vi "Teleop.vi"(10 "Match Info":T2={"Autonomous Elapsed Seconds"=0.0, "TeleOp Elapsed Seconds"=0.0, "Disabled Elapsed Seconds"=0.0, "Visited Autonomous"=FALSE, "Visited TeleOp"=FALSE, "Visited Disabled"=FALSE, "Autonomous Settings"={"Autonomous Style"=enum."Independent", "VI Refnum"=refnum}}, 11 "Call Context":T3) -> ()   [LabVIEW 2019]
doc: "This VI is called for each TeleOp packet received from the DS where the robot is not disabled. It is often used to read from the joysticks and update I/O or to update setpoints for timed control loops. It should complete and return within 20 milliseconds or it may miss DS packets."
uses:
  <vilib>/Rock Robotics/WPI/DriverStation/WPI_DriverStationDerivedRobotMode.ctl
  <vilib>/Rock Robotics/WPI/DriverStation/WPI_DriverStationMatch Info.ctl
  <vilib>/Rock Robotics/WPI/ThirdParty/Phoenix-LabVIEW/Motor Controller/Controls/CTRE_Phoenix_MotorControl_ControlMode.ctl
  <vilib>/Rock Robotics/WPI/Solenoid/WPI_SolenoidValue.ctl
  <vilib>/Rock Robotics/Network Tables/NT Read Boolean.vi
  <vilib>/Rock Robotics/Network Tables/NT Read Number.vi
  <vilib>/Rock Robotics/WPI/Utilities/WPI_GetSetVariantRefNum.vi
  <vilib>/addons/control/pid/pid.llb/PID Output Rate Limiter (DBL).vi
  <vilib>/Rock Robotics/Network Tables/NT Write Numeric Array.vi
  <vilib>/Rock Robotics/Network Tables/NT Write Boolean Array.vi
  <vilib>/Rock Robotics/WPI/Solenoid/WPI_SolenoidSetEnum.vi
  <vilib>/addons/control/pid/NI_PID_pid.lvlib
panel:
  in  "Control Panel":T1 items=["PercentOutput"=0, "Position"=1, "Velocity"=2, "Current"=3, "Follower"=5, "MotionProfile"=6, "MotionMagic"=7, "MotionProfileArc"=10, "Disabled"=15]
  in  "Climber":T1 items=["PercentOutput"=0, "Position"=1, "Velocity"=2, "Current"=3, "Follower"=5, "MotionProfile"=6, "MotionMagic"=7, "MotionProfileArc"=10, "Disabled"=15]
  in  "Outtake":T1 items=["PercentOutput"=0, "Position"=1, "Velocity"=2, "Current"=3, "Follower"=5, "MotionProfile"=6, "MotionMagic"=7, "MotionProfileArc"=10, "Disabled"=15]
  in  "Intake":T1 items=["PercentOutput"=0, "Position"=1, "Velocity"=2, "Current"=3, "Follower"=5, "MotionProfile"=6, "MotionMagic"=7, "MotionProfileArc"=10, "Disabled"=15]
  out "Sample Slider 0":dbl(slide) scale=0.0..5.0
  out "Sample Boolean 1":bool
  out "Sample Boolean 0":bool
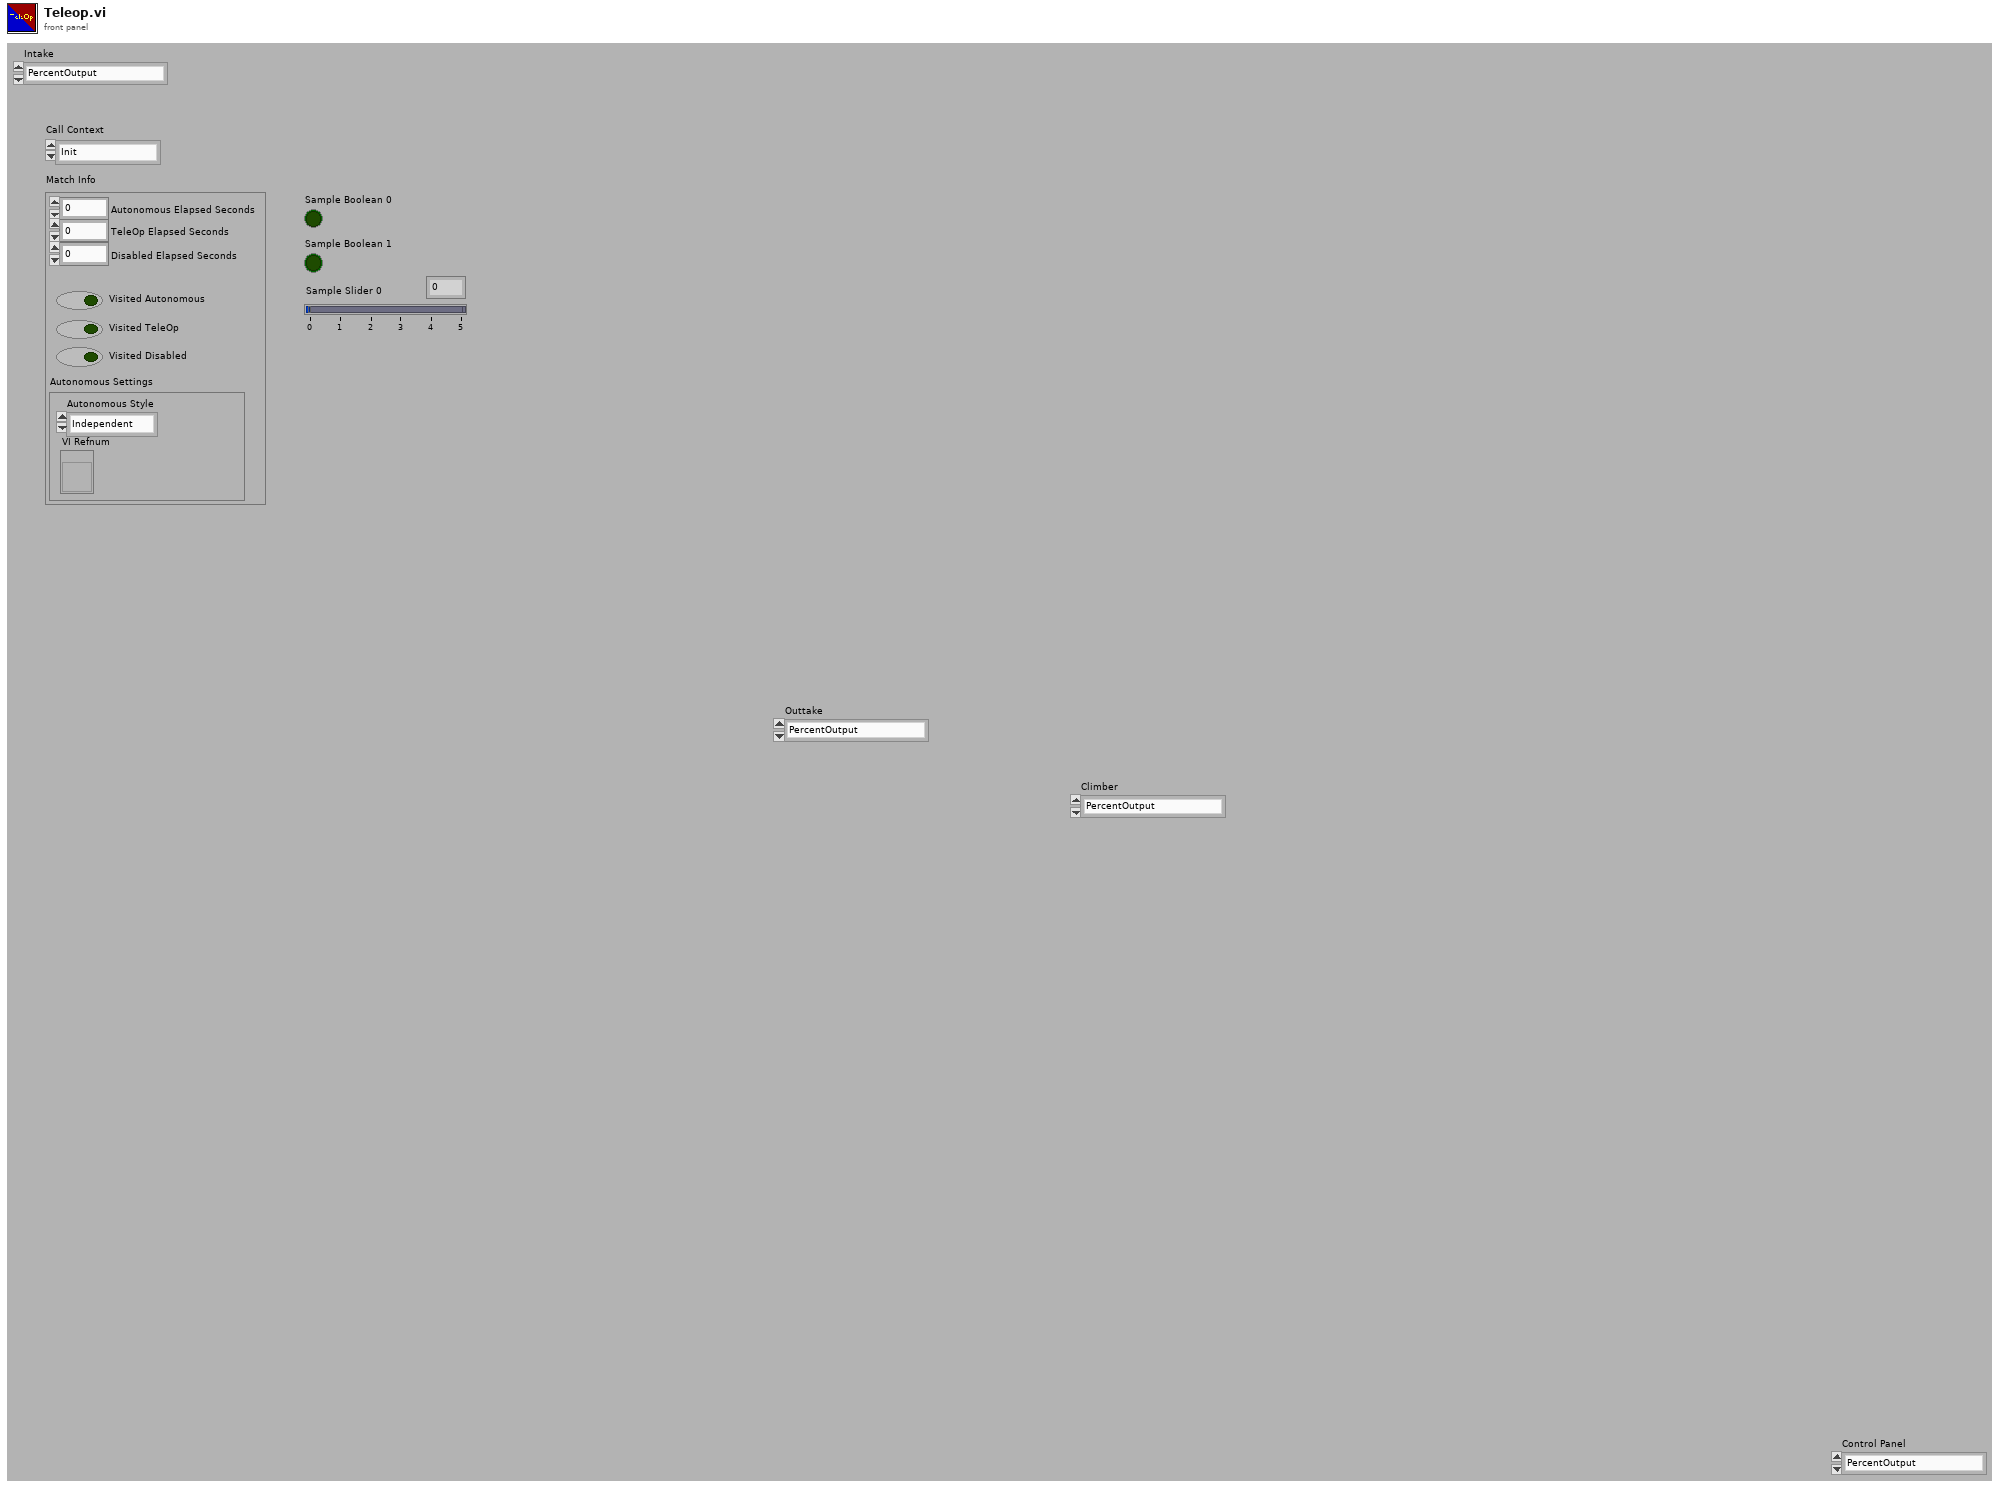
[diagram p1: front panel]
types:
  T1 = typedef "CTRE_Phoenix_MotorControl_ControlMode.ctl" = u16
  T2 = typedef "WPI_DriverStationMatch Info.ctl" = cluster{"Autonomous Elapsed Seconds":dbl, "TeleOp Elapsed Seconds":dbl, "Disabled Elapsed Seconds":dbl, "Visited Autonomous":bool, "Visited TeleOp":bool, "Visited Disabled":bool, "Autonomous Settings":cluster{"Autonomous Style":enum16{"Iterative", "Independent"}, "VI Refnum":refnum<vi>}}
  T3 = typedef "WPI_DriverStationDerivedRobotMode.ctl" = enum16{"Init", "Execute", "Stop"}
  T4 = typedef "WPI_SolenoidValue.ctl" = enum16{"Off", "On", "Forward", "Reverse"}
  T5 = typedef "WPI_RobotDriveDevRef.ctl" = cluster{"DevStatus":errorcluster, "Motors[]":T6[], "Square Inputs":bool, "Max Output":dbl}
  T6 = typedef "WPI_MotorControlDeviceRef.ctl" = cluster{"DeviceStatus":errorcluster, "Type":T7, "PWM":cluster{"PWM Channel":T8, "DeadBand":T9}, "CAN":cluster{"Device Number":u8, "SetOutput VI Ref":variant, "GetOutput VI Ref":variant, "Enable VI Ref":variant, "Disable VI Ref":variant, "Data":variant}, "Invert":bool, "DIO PWM":cluster{"PWM \"Enable\" Channel":T8, "DIOChannel":T10, "PWM Rate":dbl}}
  T7 = typedef "WPI_MotorControlType.ctl" = enum16{"PWM", "CAN", "DIO PWM"}
  T8 = typedef "FPGA_DIOPWMChannel.ctl" = enum8{"PWM 0", "PWM 1", "PWM 2", "PWM 3", "PWM 4", "PWM 5", "PWM 6", "PWM 7", "PWM 8", "PWM 9", "PWM MXP 0", "PWM MXP 1", "PWM MXP 2", "PWM MXP 3", "PWM MXP 4", "PWM MXP 5", "PWM MXP 6", "PWM MXP 7", "PWM MXP 8", "PWM MXP 9", "Invalid"}
  T9 = typedef "WPI_PWMDeadband.ctl" = cluster{"Name":string, "maxPositivePwm":i32, "minPositivePwm":i32, "centerPwm":i32, "maxNegativePwm":i32, "minNegativePwm":i32, "angularRange":u16}
  T10 = typedef "FPGA_DIOChannel.ctl" = enum8{"DIO 0", "DIO 1", "DIO 2", "DIO 3", "DIO 4", "DIO 5", "DIO 6", "DIO 7", "DIO 8", "DIO 9", "DIO MXP 0", "DIO MXP 1", "DIO MXP 2", "DIO MXP 3", "DIO MXP 4", "DIO MXP 5", "DIO MXP 6", "DIO MXP 7", "DIO MXP 8", "DIO MXP 9", "DIO MXP 10", "DIO MXP 11", "DIO MXP 12", "DIO MXP 13", "DIO MXP 14", "DIO MXP 15", "SPI Port CS1", "SPI Port CS2", "SPI Port CS3", "SPI Port MISO", "SPI Port MOSI", "Invalid"}
  T11 = typedef "WPI_JoystickDevRef.ctl" = cluster{"Device":T12}
  T12 = typedef "WPI_JoystickDeviceEnum.ctl" = enum16{"USB 0", "USB 1", "USB 2", "USB 3", "USB 4", "USB 5"}
  T13 = typedef "WPI_SolenoidDevRef.ctl" = cluster{"DevStatus":errorcluster, "Pneumatics Control Module":u8, "Forward Solenoid Channel":T14, "Reverse Solenoid Channel":T14}
  T14 = typedef "WPI_SolenoidChannel.ctl" = enum8{"Solenoid 0", "Solenoid 1", "Solenoid 2", "Solenoid 3", "Solenoid 4", "Solenoid 5", "Solenoid 6", "Solenoid 7", "Invalid"}
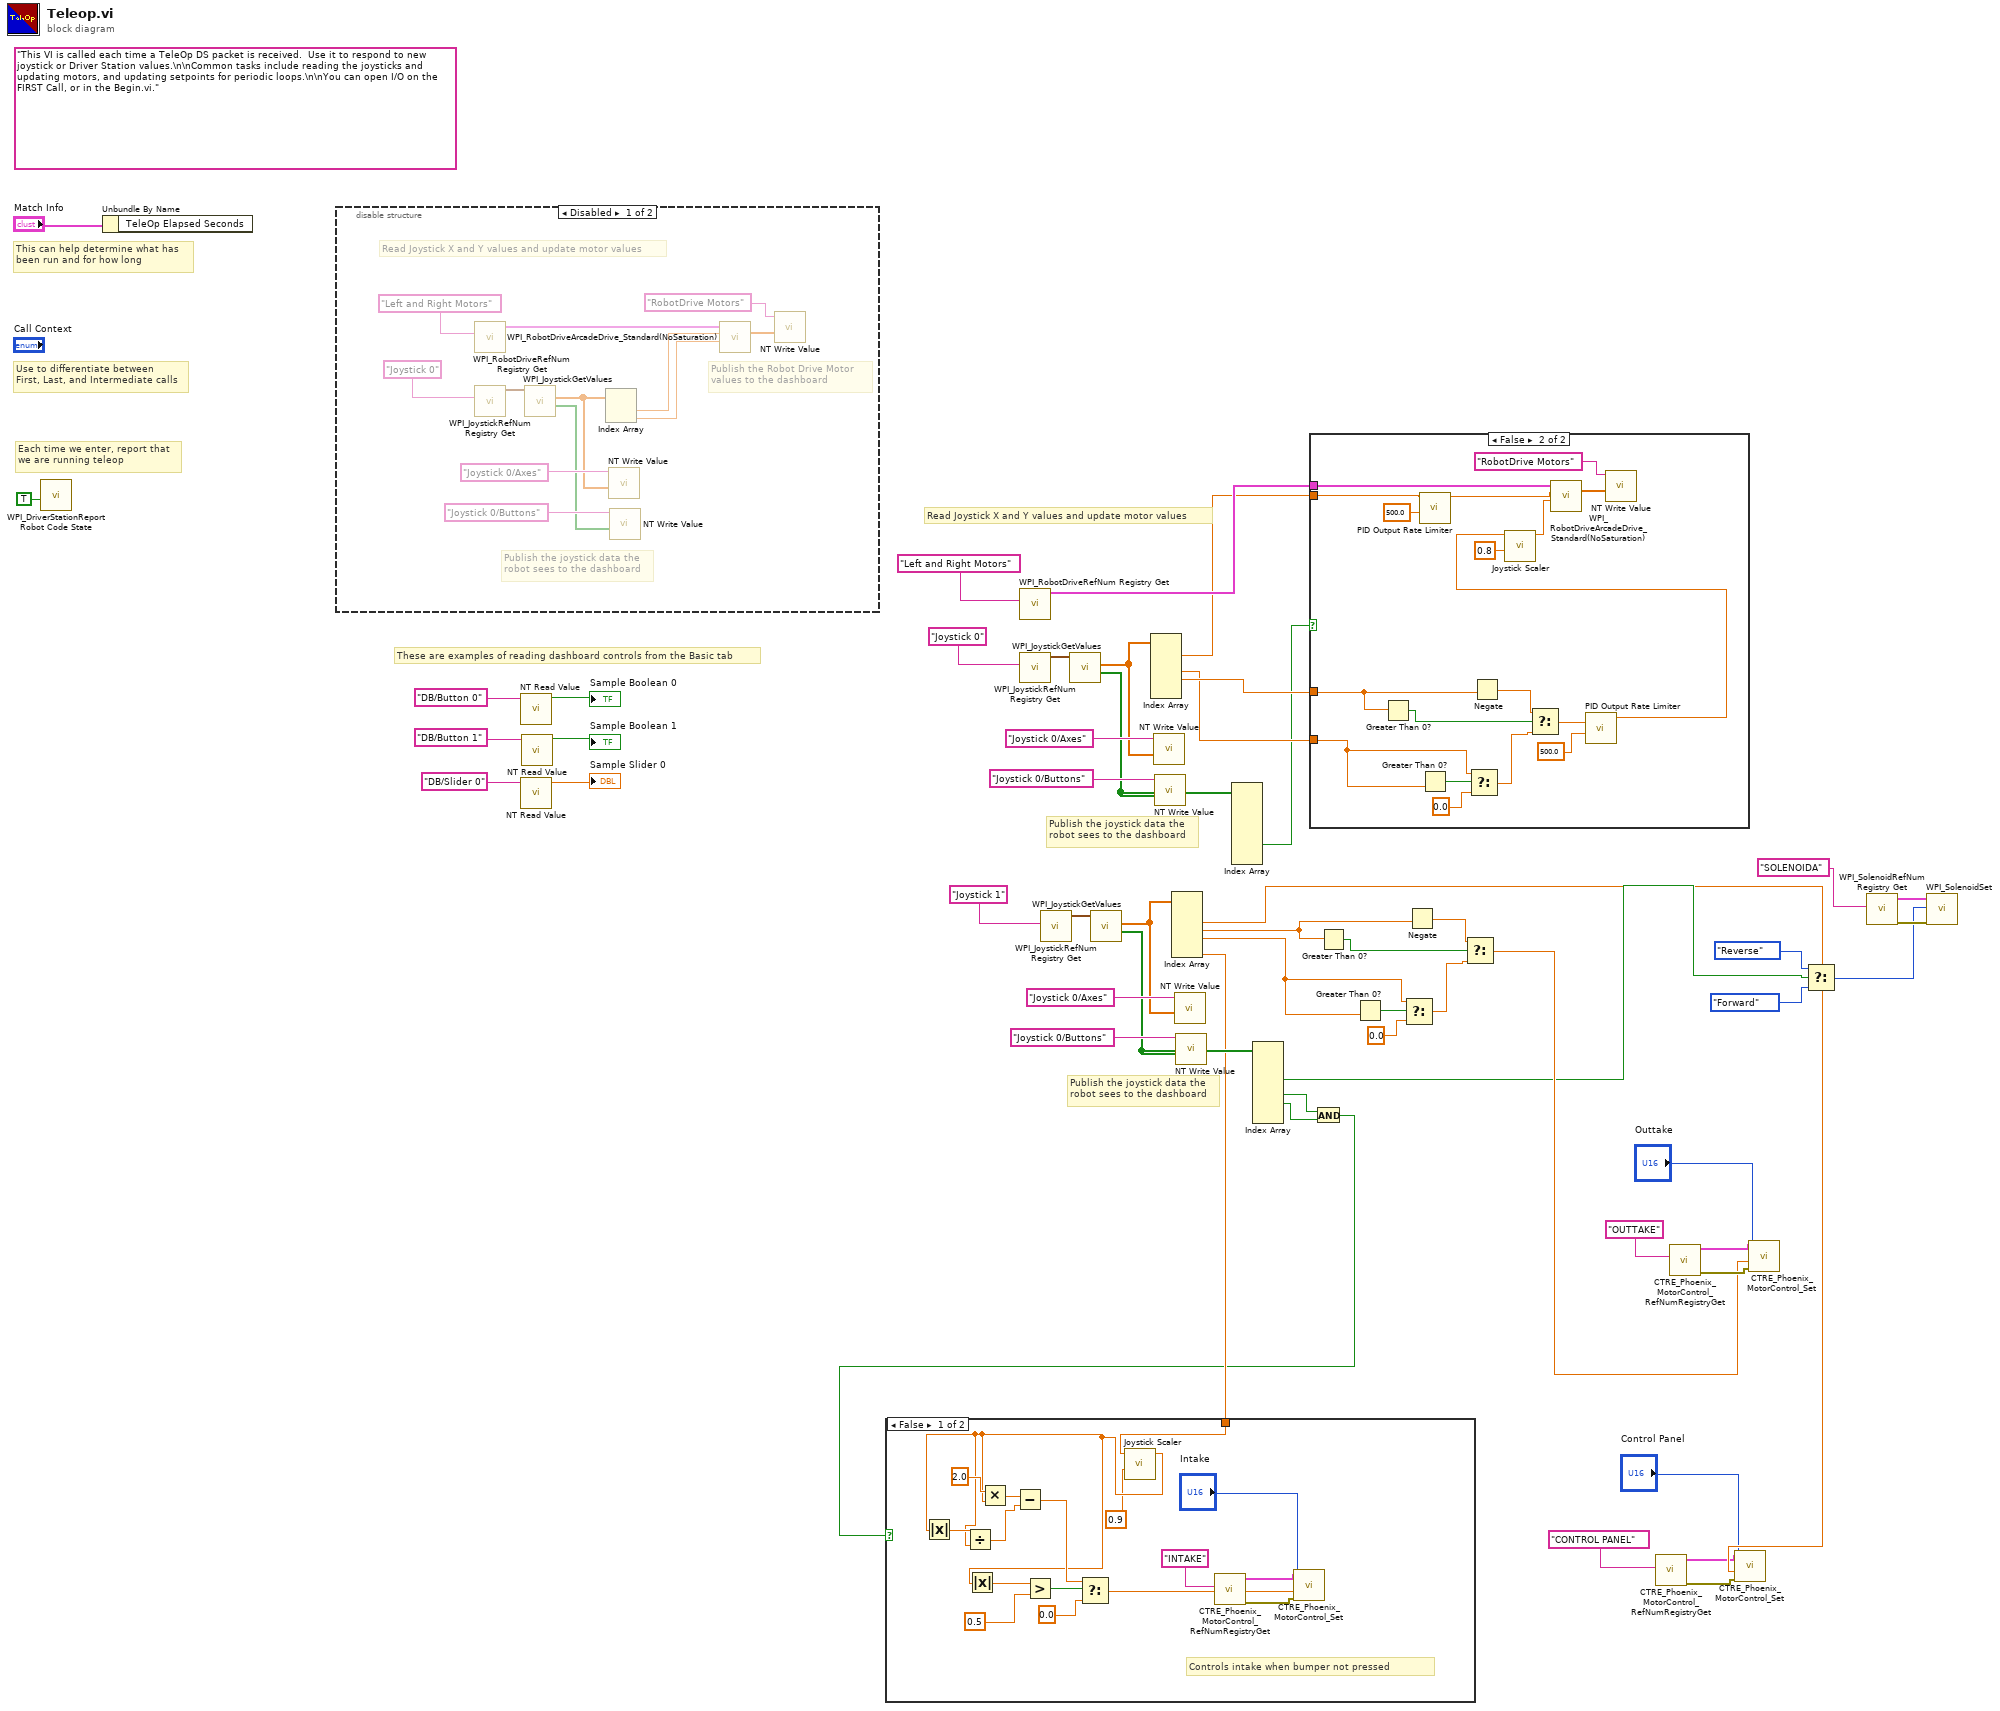
[diagram p0: block diagram]
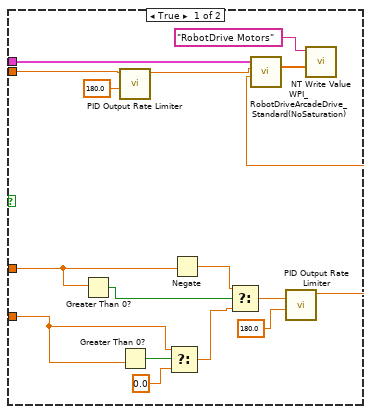
[diagram p2: hidden frame]
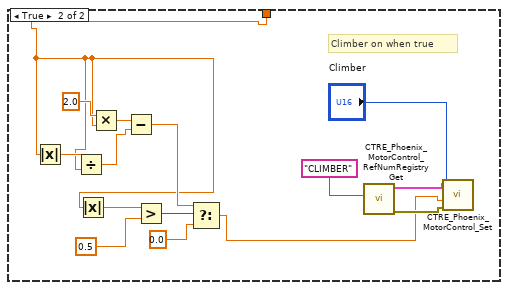
[diagram p3: hidden frame]
diagram:
  (unwired) "This VI is called each time a TeleOp DS packet is received.  Use it to respond to new joystick or Driver Station values.\n\nCommon tasks include reading the joysticks and updating motors, and updating setpoints for periodic loops.\n\nYou can open I/O on the FIRST Call, or in the Begin.vi."
  # "Publish the joystick data the\nrobot sees to the dashboard"
  # "Publish the joystick data the\nrobot sees to the dashboard"
  # "Read Joystick X and Y values and update motor values"
  # "These are examples of reading dashboard controls from the Basic tab"
  # "Each time we enter, report that\nwe are running teleop"
  # "Use to differentiate between\nFirst, Last, and Intermediate calls"
  # "This can help determine what has\nbeen run and for how long"
  n1 = call <vilib>:"WPI_DriverStationReport Robot Code State.vi"("TeleOp"=TRUE ("Autonomous")) -> ()  [unwired: 10 in, 1 out]
  n2 = Unbundle By Name("Match Info") -> ()  [unwired: 1 out]
  n3 = disable-structure shown="Disabled" {
    frame Disabled {
      # "Publish the Robot Drive Motor\nvalues to the dashboard"
      # "Publish the joystick data the\nrobot sees to the dashboard"
      # "Read Joystick X and Y values and update motor values"
      n4 = call <vilib>:"WPI_RobotDriveRefNum Registry Get.vi"("refnum name"="Left and Right Motors") -> ("RobotDriveDevRef"=w65:T5)  [unwired: 1 in, 9 out]
      n5 = call <vilib>:"WPI_JoystickRefNum Registry Get.vi"("refnum name"="Joystick 0") -> ("JoystickDevRef"=w62:T11)  [unwired: 1 in, 9 out]
      n6 = call <vilib>:"WPI_JoystickGetValues.vi"("JoystickDevRef"=w62) -> ("Buttons"=w57:bool[], "Axes"=w58:dbl[])  [unwired: 6 in, 3 out]
      n7 = Index Array(array=w58) -> (element #1=w64:dbl, element #2=w61:dbl)  [unwired: 2 in]
      n8 = call-poly <vilib>:"NT Write Value.vi"("Numeric Array"=w58, "Name"="Joystick 0/Axes") -> ()  [unwired: 9 in, 1 out]
      n9 = call-poly <vilib>:"NT Write Value.vi"("Boolean Array"=w57, "Name"="Joystick 0/Buttons") -> ()  [unwired: 9 in, 1 out]
      n10 = call <vilib>:"WPI_RobotDriveArcadeDrive_Standard(NoSaturation).vi"("Y axis value"=w61, "X axis value"=w64, "RobotDriveDevRef"=w65) -> ("Motor Values"=w56:dbl[])  [unwired: 1 in, 7 out]
      n11 = call-poly <vilib>:"NT Write Value.vi"("Numeric Array"=w56, "Name"="RobotDrive Motors") -> ()  [unwired: 9 in, 1 out]
    }
    frame Enabled {
    }
  }
  n12 = call-poly <vilib>:"NT Read Value.vi"("Name"="DB/Button 0" ("refnum name")) -> ("Boolean"=→"Sample Boolean 0":bool)  [unwired: 9 in, 1 out]
  n13 = call-poly <vilib>:"NT Read Value.vi"("Name"="DB/Slider 0" ("refnum name")) -> ("Numeric"=→"Sample Slider 0":dbl)  [unwired: 9 in, 1 out]
  n14 = call-poly <vilib>:"NT Read Value.vi"("Name"="DB/Button 1" ("refnum name")) -> ("Boolean"=→"Sample Boolean 1":bool)  [unwired: 9 in, 1 out]
  n15 = call <vilib>:"WPI_RobotDriveRefNum Registry Get.vi"("refnum name"="Left and Right Motors") -> ("RobotDriveDevRef"=w39:T5)  [unwired: 1 in, 9 out]
  n16 = call <vilib>:"WPI_JoystickRefNum Registry Get.vi"("refnum name"="Joystick 0") -> ("JoystickDevRef"=w44:T11)  [unwired: 1 in, 9 out]
  n17 = call <vilib>:"WPI_JoystickRefNum Registry Get.vi"("refnum name"="Joystick 1") -> ("JoystickDevRef"=w26:T11)  [unwired: 1 in, 9 out]
  n18 = call <vilib>:"WPI_JoystickGetValues.vi"("JoystickDevRef"=w44) -> ("Buttons"=w40:bool[], "Axes"=w41:dbl[])  [unwired: 6 in, 3 out]
  n19 = call <vilib>:"WPI_JoystickGetValues.vi"("JoystickDevRef"=w26) -> ("Buttons"=w22:bool[], "Axes"=w23:dbl[])  [unwired: 6 in, 3 out]
  n20 = Index Array(array=w41) -> (element #1=w11:dbl, element #3=w2:dbl, element #4=w32:dbl)  [unwired: 6 in, 3 out]
  n21 = call-poly <vilib>:"NT Write Value.vi"("Numeric Array"=w41, "Name"="Joystick 0/Axes") -> ()  [unwired: 9 in, 1 out]
  n22 = call-poly <vilib>:"NT Write Value.vi"("Boolean Array"=w40, "Name"="Joystick 0/Buttons") -> ()  [unwired: 9 in, 1 out]
  n23 = Index Array(array=w23) -> (element #2=w12:dbl, element #3=w14:dbl, element #4=w15:dbl, element #6=w6:dbl)  [unwired: 6 in, 2 out]
  n24 = call-poly <vilib>:"NT Write Value.vi"("Numeric Array"=w23, "Name"="Joystick 0/Axes") -> ()  [unwired: 9 in, 1 out]
  n25 = call-poly <vilib>:"NT Write Value.vi"("Boolean Array"=w22, "Name"="Joystick 0/Buttons") -> ()  [unwired: 9 in, 1 out]
  n26 = Index Array(array=w40) -> (element #6=w1:bool)  [unwired: 8 in, 7 out]
  n27 = Index Array(array=w22) -> (element #3=w13:bool, element #5=w5:bool, element #6=w4:bool)  [unwired: 8 in, 5 out]
  n28 = case shown="False" w1 {
    tunnel: w39 -> [w82 w100]
    tunnel: w32 -> [w76 w94]
    tunnel: w11 -> [w72 w90]
    tunnel: w2 -> [w67 w86]
    frame True {
      n29 = Greater Than 0?(x=w76) -> (x > 0?=w81:bool)
      n30 = call-poly <vilib>:"PID Output Rate Limiter.vi"("output rate (EGU/min)"=180.0, "input (controller output)"=w72) -> ("output"=w71:dbl)  [unwired: 6 in, 1 out]
      n31 = Greater Than 0?(x=w67) -> (x > 0?=w79:bool)
      n32 = Select(t=w67, s=w79, f=0.0) -> (s? t:f=w77:dbl)
      n33 = Negate(x=w76) -> (-x=w80:dbl)
      n34 = Select(t=w80, s=w81, f=w77) -> (s? t:f=w73:dbl)
      n35 = call-poly <vilib>:"PID Output Rate Limiter.vi"("output rate (EGU/min)"=180.0, "input (controller output)"=w73) -> ("output"=w68:dbl)  [unwired: 6 in, 1 out]
      n36 = call <vilib>:"WPI_RobotDriveArcadeDrive_Standard(NoSaturation).vi"("Y axis value"=w68, "X axis value"=w71, "RobotDriveDevRef"=w82) -> ("Motor Values"=w75:dbl[])  [unwired: 1 in, 7 out]
      n37 = call-poly <vilib>:"NT Write Value.vi"("Numeric Array"=w75, "Name"="RobotDrive Motors") -> ()  [unwired: 9 in, 1 out]
    }
    frame False {
      n38 = Greater Than 0?(x=w94) -> (x > 0?=w99:bool)
      n39 = call-poly <vilib>:"PID Output Rate Limiter.vi"("output rate (EGU/min)"=500.0, "input (controller output)"=w90) -> ("output"=w89:dbl)  [unwired: 6 in, 1 out]
      n40 = Greater Than 0?(x=w86) -> (x > 0?=w97:bool)
      n41 = Select(t=w86, s=w97, f=0.0) -> (s? t:f=w95:dbl)
      n42 = Negate(x=w94) -> (-x=w98:dbl)
      n43 = Select(t=w98, s=w99, f=w95) -> (s? t:f=w91:dbl)
      n44 = call-poly <vilib>:"PID Output Rate Limiter.vi"("output rate (EGU/min)"=500.0, "input (controller output)"=w91) -> ("output"=w84:dbl)  [unwired: 6 in, 1 out]
      n45 = call "Joystick Scaler.vi"("Scaler"=0.8, "Joystick Value"=w84) -> ("Final Joystick Value"=w83:dbl)  [unwired: 9 in]
      n46 = call <vilib>:"WPI_RobotDriveArcadeDrive_Standard(NoSaturation).vi"("Y axis value"=w83, "X axis value"=w89, "RobotDriveDevRef"=w100) -> ("Motor Values"=w93:dbl[])  [unwired: 1 in, 7 out]
      n47 = call-poly <vilib>:"NT Write Value.vi"("Numeric Array"=w93, "Name"="RobotDrive Motors") -> ()  [unwired: 9 in, 1 out]
    }
  }
  n48 = And(x=w5, y=w4) -> (x .and. y?=w3:bool)
  n49 = case shown="False" w3 {
    tunnel: w6 -> [w102 w119]
    frame False {
      # "Controls intake when bumper not pressed"
      n50 = call "Joystick Scaler.vi"("Scaler"=0.9, "Joystick Value"=w102) -> ("Final Joystick Value"=w103:dbl)  [unwired: 9 in]
      n51 = Absolute Value(x=w103) -> (abs(x)=w117:dbl)
      n52 = Divide(x=w117, y=w103) -> (x/y=w116:dbl)
      n53 = Absolute Value(x=w103) -> (abs(x)=w111:dbl)
      n54 = Multiply(x=2.0, y=w103) -> (x*y=w114:dbl)
      n55 = Subtract(x=w114, y=w116) -> (x-y=w115:dbl)
      n56 = Greater?(x=w111, y=0.5) -> (0:w112:bool)
      n57 = Select(t=w115, s=w112, f=0.0) -> (s? t:f=w113:dbl)
      n58 = call <vilib>:"CTRE_Phoenix_MotorControl_RefNumRegistryGet.vi"("refnum name"="INTAKE") -> ("error out"=w109:errorcluster, "PhoenixMotorControlDevRef"=w108:T6)  [unwired: 9 in]
      n59 = call <vilib>:"CTRE_Phoenix_MotorControl_Set.vi"("error in (no error)"=w109, "Output"=w113, "Control Mode"="Intake", "PhoenixMotorControlDevRef"=w108) -> ()  [unwired: 6 in, 2 out]
    }
    frame True {
      # "Climber on when true"
      n60 = Absolute Value(x=w119) -> (abs(x)=w128:dbl)
      n61 = Divide(x=w128, y=w119) -> (x/y=w127:dbl)
      n62 = Absolute Value(x=w119) -> (abs(x)=w123:dbl)
      n63 = Multiply(x=2.0, y=w119) -> (x*y=w125:dbl)
      n64 = Subtract(x=w125, y=w127) -> (x-y=w126:dbl)
      n65 = Greater?(x=w123, y=0.5) -> (0:w124:bool)
      n66 = Select(t=w126, s=w124, f=0.0) -> (s? t:f=w118:dbl)
      n67 = call <vilib>:"CTRE_Phoenix_MotorControl_RefNumRegistryGet.vi"("refnum name"="CLIMBER") -> ("error out"=w130:errorcluster, "PhoenixMotorControlDevRef"=w131:T6)  [unwired: 9 in]
      n68 = call <vilib>:"CTRE_Phoenix_MotorControl_Set.vi"("error in (no error)"=w130, "Output"=w118, "Control Mode"="Climber", "PhoenixMotorControlDevRef"=w131) -> ()  [unwired: 6 in, 2 out]
    }
  }
  n69 = Greater Than 0?(x=w14) -> (x > 0?=w21:bool)
  n70 = Greater Than 0?(x=w15) -> (x > 0?=w19:bool)
  n71 = Select(t=w15, s=w19, f=0.0) -> (s? t:f=w17:dbl)
  n72 = Negate(x=w14) -> (-x=w20:dbl)
  n73 = Select(t=w20, s=w21, f=w17) -> (s? t:f=w16:dbl)
  n74 = call <vilib>:"CTRE_Phoenix_MotorControl_RefNumRegistryGet.vi"("refnum name"="CONTROL PANEL") -> ("error out"=w8:errorcluster, "PhoenixMotorControlDevRef"=w9:T6)  [unwired: 9 in]
  n75 = call <vilib>:"CTRE_Phoenix_MotorControl_RefNumRegistryGet.vi"("refnum name"="OUTTAKE") -> ("error out"=w29:errorcluster, "PhoenixMotorControlDevRef"=w30:T6)  [unwired: 9 in]
  n76 = call <vilib>:"CTRE_Phoenix_MotorControl_Set.vi"("error in (no error)"=w8, "Output"=w12, "Control Mode"="Control Panel", "PhoenixMotorControlDevRef"=w9) -> ()  [unwired: 6 in, 2 out]
  n77 = call <vilib>:"CTRE_Phoenix_MotorControl_Set.vi"("error in (no error)"=w29, "Output"=w16, "Control Mode"="Outtake", "PhoenixMotorControlDevRef"=w30) -> ()  [unwired: 6 in, 2 out]
  n78 = Select(t=WPI_SolenoidValue."Reverse" ("Value"), s=w13, f=WPI_SolenoidValue."Forward" ("Value")) -> (s? t:f=w35:T4)
  n79 = call <vilib>:"WPI_SolenoidRefNum Registry Get.vi"("refnum name"="SOLENOIDA") -> ("error out"=w38:errorcluster, "SolenoidDevRef"=w37:T13)  [unwired: 9 in]
  n80 = call-poly <vilib>:"WPI_SolenoidSet.vi"("error in (no error)"=w38, "Value"=w35, "SolenoidDevRef"=w37) -> ()  [unwired: 7 in, 2 out]
